vi "CreateBurstModeDataEvent.vi"(7 "Qbus in":refnum<class "Qbus.lvclass">, 8 "error in (no error)":errorcluster, 10 "data":T2, 11 "config":T1) -> (0 "error out":errorcluster, 3 "config out":T1)   [LabVIEW 2017, in "CmsDataEventCreator.lvlib"]
uses:
  <vilib>/addons/InsightCM/Devices/Shared/Cms/CmsDataEventCreator/CmsDataEventCreator.lvlib
  <vilib>/addons/InsightCM/Devices/Shared/Common/DataFlow/controls/Data.ctl
  <vilib>/addons/InsightCM/Utilities/DataAccessors/controls/wfmSGL_DVR.ctl
  <vilib>/addons/PointValueMap/controls/PointMap.ctl
  <vilib>/addons/InsightCM/Devices/Shared/Common/DataFlow/controls/Type.ctl
  <vilib>/addons/Qbus/Qbus.lvclass
  <vilib>/addons/InsightCM/Devices/Shared/Cms/CmsDataEventCreator/controls/config.ctl
  <vilib>/addons/InsightCM/Devices/Shared/Cms/CmsDataEventCreator/controls/DataEventConfig.ctl
  <vilib>/addons/InsightCM/Devices/Shared/Cms/CmsDataEventCreator/controls/AcqParams.ctl
  <vilib>/addons/InsightCM/Devices/Shared/Common/DataAccumulator/controls/AccumulationSettings.ctl
  <vilib>/addons/InsightCM/Devices/Shared/Common/DataAccumulator/controls/accumulationType.ctl
  <vilib>/addons/InsightCM/Devices/Shared/Common/DVRBuffer/controls/BufferLocation.ctl
  <vilib>/addons/PointValueMap/subVIs/Point_Read_string.vi
  <vilib>/addons/InsightCM/Devices/Shared/Common/DataAccumulator/DataAccumulator.lvlib
  <vilib>/addons/InsightCM/Devices/Shared/Common/DVRBuffer/DVRBuffer.lvlib
  <vilib>/addons/PointValueMap/PointValueMap.lvlib
  <vilib>/addons/InsightCM/Devices/Shared/Common/DataFlow/DataFlow.lvlib
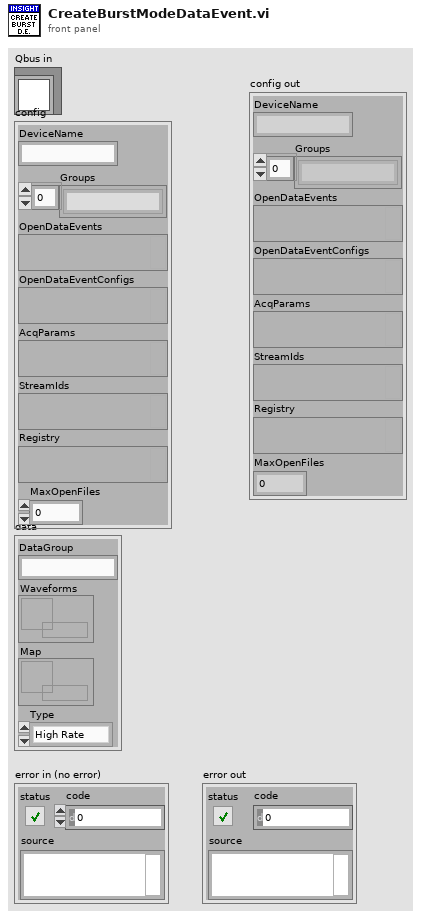
[diagram p1: front panel]
types:
  T1 = typedef "CmsDataEventCreator.lvlib/config.ctl" = cluster{"DeviceName":string, "Groups":string[], "OpenDataEvents":variant, "OpenDataEventConfigs":variant, "AcqParams":variant, "StreamIds":variant, "Registry":variant, "MaxOpenFiles":i32}
  T2 = typedef "DataFlow.lvlib/Data.ctl" = cluster{"DataGroup":string, "Waveforms":T3, "Map":T4, "Type":T5}
  T3 = typedef "wfmSGL_DVR.ctl" = refnum<data-value>
  T4 = typedef "PointValueMap.lvlib/PointMap.ctl" = refnum<data-value>
  T5 = typedef "DataFlow.lvlib/Type.ctl" = enum16{"High Rate", "Low Rate", "Burst Mode"}
  T6 = typedef "CmsDataEventCreator.lvlib/DataEventConfig.ctl" = cluster{"AcqParams":T7, "OpState":string, "ExitOpState":bool, "Reason":string, "StreamId":string, "Map":T4, "DataSetIds":variant, "IncludeWaveforms":bool, "TrendPointsOnly":bool}
  T7 = typedef "CmsDataEventCreator.lvlib/AcqParams.ctl" = cluster{"Stream":bool, "PreTrigger":i32, "CollectOnEnter":bool, "Enter PreTrigger":i32, "Enter Length":dbl, "CollectOnExit":bool, "ContinuousData":bool, "Accumulation Settings":T8}
  T8 = typedef "DataAccumulator.lvlib/AccumulationSettings.ctl" = cluster{"Type":T9, "Length":dbl, "Max Time (sec)":dbl, "Start Block":T10, "Acquired (sec)":dbl, "Acquired (pulses)":i32, "Initial Pulse Offset":dbl, "Stop Block":T10, "LastBlockAdded":u32}
  T9 = typedef "DataAccumulator.lvlib/accumulationType.ctl" = enum16{"none", "seconds", "revolutions"}
  T10 = typedef "DVRBuffer.lvlib/BufferLocation.ctl" = cluster{"Block":u32, "Index":i32}
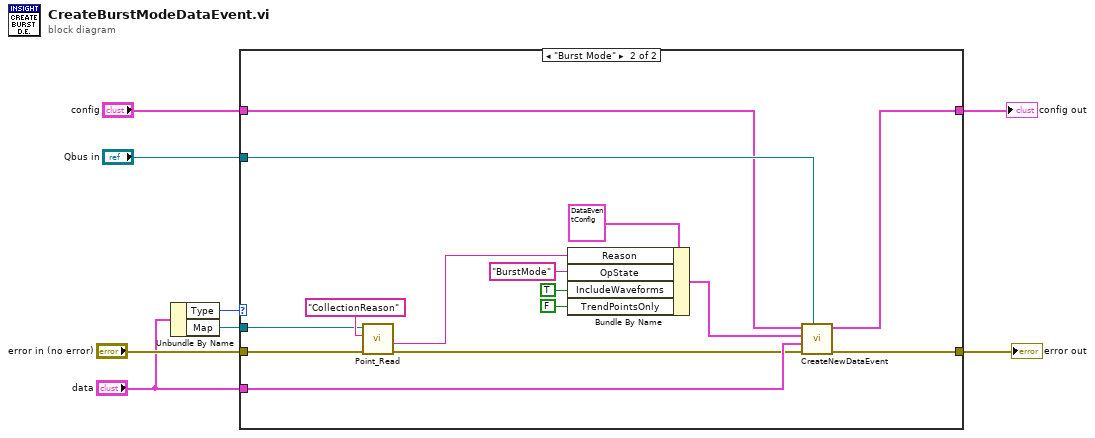
[diagram p0: block diagram]
diagram:
  n1 = Unbundle By Name("data") -> ("Type"=w1:T5, "Map"=w2:T4)
  n2 = case shown="\"Burst Mode\"" w1 {
    tunnel: "error in (no error)" -> [w9 w13]
    tunnel: "Qbus in" -> [_ w25]
    tunnel: [w10 w24] -> w6
    tunnel: "config" -> [w10 w23]
    tunnel: [w9 w22] -> w4
    tunnel: "data" -> [_ w20]
    tunnel: w2 -> [_ w14]
    frame Default {
    }
    frame "Burst Mode" {
      n3 = call-poly <vilib>:"Point_Read.vi"("Error In"=w13, "Tag"="CollectionReason", "Map"=w14) -> ("Error Out"=w12:errorcluster, "Value"=w11:string)  [unwired: 3 in, 4 out]
      n4 = Bundle By Name(cluster=T6 {"AcqParams"={"Stream"=FALSE, "PreTrigger"=0, "CollectOnEnter"=FALSE, "Enter PreTrigger"=0, "Enter Length"=0.0, "CollectOnExit"=FALSE, "ContinuousData"=FALSE, "Accumulation Settings"={"Type"=enum."none", "Length"=0.0, "Max Time (sec)"=0.0, "Start Block"={"Block"=0, "Index"=0}, "Acquired (sec)"=0.0, "Acquired (pulses)"=0, "Initial Pulse Offset"=0.0, "Stop Block"={"Block"=0, "Index"=0}, "LastBlockAdded"=0}}, "OpState"="", "ExitOpState"=FALSE, "Reason"="", "StreamId"="", "Map"=refnum, "DataSetIds"=variant, "IncludeWaveforms"=FALSE, "TrendPointsOnly"=FALSE} ("data event config"), "Reason"=w11, "OpState"="BurstMode" ("Reason"), "IncludeWaveforms"=TRUE, "TrendPointsOnly"=FALSE) -> (w17:T6)
      n5 = call <vilib>:"CreateNewDataEvent.vi"("Qbus"=w25, "error in (no error)"=w12, "data flow"=w20, "data event config"=w17, "config"=w23) -> ("error out"=w22:errorcluster, "config out"=w24:T1)  [unwired: 5 in]
    }
  }
  "config out" <- w6
  "error out" <- w4
